vi "WM Check Limits.vi"(0 "Input Time Series":dbl[](array[numeric]) format="%.2f", 1 "Sampling Rate (Hz)":dbl format="%.2f", 2 "Limit Settings":T1={"Min Wave Period"=0.9, "Max Wave Period"=5.0, "Cutoff Frequency"=2.0, "Max 1/2 Piston Stroke"=0.16, "Max H/L"=0.1, "Max H/d"=0.65} {"Max H/d" format="%.2f"; "Max H/L" format="%.2f"; "Max 1/2 Piston Stroke" format="%.2f"; "Cutoff Frequency" format="%.2f"; "Max Wave Period" format="%.2f"; "Min Wave Period" format="%.2f"}, 3 "Water Depth (m)":dbl format="%.2f", 4 "Paddle Height (m)":dbl=3.3147 format="%.4f") -> (5 "Wave Period OK":bool, 6 "Wave Height OK":bool, 7 "Error Message":string, 8 "Significant Wave Height (m)":dbl format="%.2f", 9 "Significant Wave Period (s)":dbl format="%.2f")   [LabVIEW 2012]
panel:
  # "m"
  # "s"
  # "s"
  # "Hz"
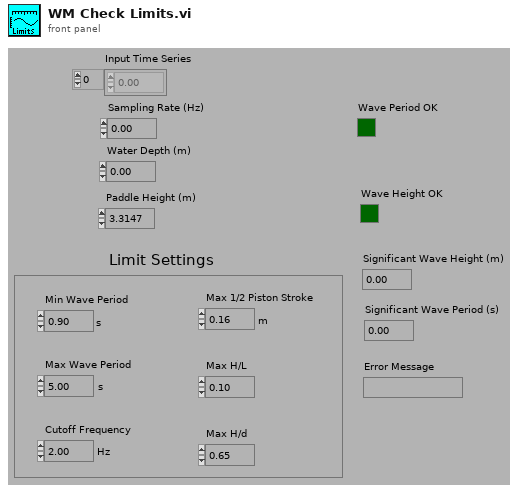
[diagram p1: front panel]
types:
  T1 = cluster{"Min Wave Period":dbl, "Max Wave Period":dbl, "Cutoff Frequency":dbl, "Max 1/2 Piston Stroke":dbl, "Max H/L":dbl, "Max H/d":dbl}
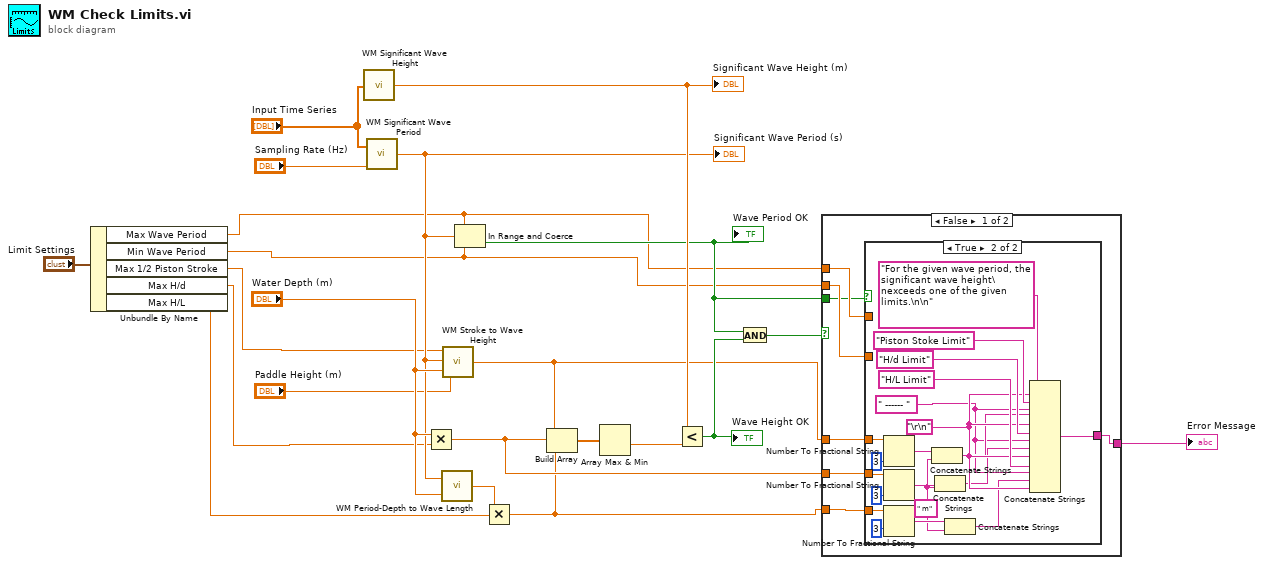
[diagram p0: block diagram]
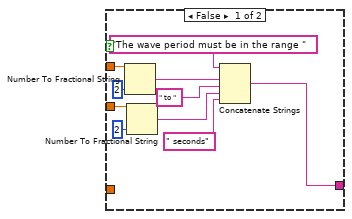
[diagram p2: hidden frame]
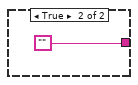
[diagram p3: hidden frame]
diagram:
  n1 = Unbundle By Name("Limit Settings") -> ("Max Wave Period"=w5:dbl, "Min Wave Period"=w4:dbl, "Max 1/2 Piston Stroke"=w3:dbl, "Max H/d"=w2:dbl, "Max H/L"=w1:dbl)
  n2 = call "WM Significant Wave Height.vi"("Input"="Input Time Series") -> ("Significant Wave Height"=w16:dbl)
  "Significant Wave Height (m)" <- w16
  n3 = call "WM Significant Wave Period.vi"("Sampling Rate"="Sampling Rate (Hz)", "Time Series"="Input Time Series") -> ("Significant Wave Period"=w15:dbl)
  "Significant Wave Period (s)" <- w15
  n4 = Multiply(x="Water Depth (m)", y=w2) -> (x*y=w10:dbl)
  n5 = call "WM Period-Depth to Wave Length.vi"("Water Depth"="Water Depth (m)", "Period"=w15) -> ("WaveLength"=w19:dbl)
  n6 = call "WM Stroke to Wave Height.vi"("Paddle Height (m)"="Paddle Height (m)", "Wave Period (s)"=w15, "Water Depth (m)"="Water Depth (m)", "Flap Amplitude from x=0 (m)"=w3) -> ("Wave Height (m)"=w11:dbl)
  n7 = In Range and Coerce(upper limit=w5, x=w15, lower limit=w4) -> (In Range?=w12:bool)  [unwired: 1 out]
  "Wave Period OK" <- w12
  n8 = Multiply(x=w19, y=w1) -> (x*y=w9:dbl)
  n9 = Build Array(w11, w10, w9) -> (w18:dbl[])
  n10 = Array Max & Min(array=w18) -> (min value=w17:dbl)  [unwired: 3 out]
  n11 = Less?(x=w16, y=w17) -> (x < y?=w14:bool)
  "Wave Height OK" <- w14
  n12 = And(x=w12, y=w14) -> (x .and. y?=w13:bool)
  n13 = case shown="False" w13 {
    tunnel: w5 -> [w29 _]
    tunnel: w4 -> [w28 _]
    tunnel: w12 -> [w27 _]
    tunnel: w11 -> [w26 _]
    tunnel: w10 -> [w25 _]
    tunnel: w9 -> [w24 _]
    tunnel: [w23 ""] -> w8
    frame False {
      n14 = case shown="True" w27 {
        tunnel: w29 -> [w38 _]
        tunnel: w28 -> [w37 _]
        tunnel: w26 -> [_ w59]
        tunnel: w25 -> [_ w58]
        tunnel: w24 -> [_ w57]
        tunnel: [w30 w52] -> w23
        frame False {
          n15 = Number To Fractional String(number=w38, precision (6)=i16 2) -> (F-format string=w34:string)  [unwired: 2 in]
          n16 = Number To Fractional String(number=w37, precision (6)=i16 2) -> (F-format string=w32:string)  [unwired: 2 in]
          n17 = Concatenate Strings("The wave period must be in the range ", w34, " to ", w32, " seconds" ("Substring")) -> (w30:string)
        }
        frame True {
          w40 = " ------ "
          w41 = " m"
          w47 = "\r\n"
          n18 = Number To Fractional String(number=w59, precision (6)=i16 3) -> (F-format string=w50:string)  [unwired: 2 in]
          n19 = Number To Fractional String(number=w58, precision (6)=i16 3) -> (F-format string=w44:string)  [unwired: 2 in]
          n20 = Number To Fractional String(number=w57, precision (6)=i16 3) -> (F-format string=w46:string)  [unwired: 2 in]
          n21 = Concatenate Strings(w50, w41) -> (w42:string)
          n22 = Concatenate Strings(w44, w41) -> (w43:string)
          n23 = Concatenate Strings(w46, w41) -> (w45:string)
          n24 = Concatenate Strings("For the given wave period, the significant wave height\nexceeds one of the given limits.\n\n", w47, "Piston Stoke Limit", w40, w42, w47, "H/d Limit", w40, w43, w47, "H/L Limit", w40, w45, w47) -> (w52:string)
        }
      }
    }
    frame True {
    }
  }
  "Error Message" <- w8
